vi "Sensor.vi"(0 "VISA resource name":refnum<visa-resource-name>, 7 "Channel (1)":i32=1 min=1 max=16 step=1, 11 "error in (no error)":errorcluster) -> (4 "VISA resource name out":refnum<visa-resource-name>, 6 "Resistance Reading":dbl min=0.0 max=63200000.0 step=1e-05 format="%^.5e", 8 "Kelvin Reading":dbl min=0.0 max=1000.0 step=1e-05 format="%^.5e", 10 "Power Reading":dbl min=0.0 max=0.01 step=1e-05 format="%^.5e", 15 "error out":errorcluster)   [LabVIEW 2014, in "Lake Shore Cryotronics 370.lvlib"]
doc: "This VI querys the instrument for an channels's sensor reading in Resistance, Kelvin, and Power."
uses:
  Lake Shore Cryotronics 370.lvlib
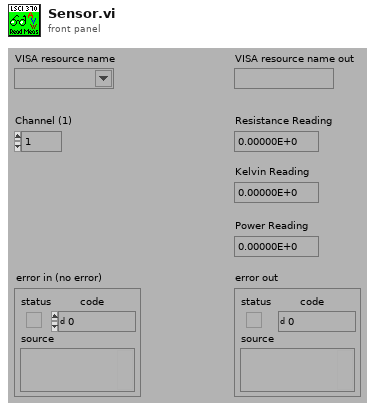
[diagram p1: front panel]
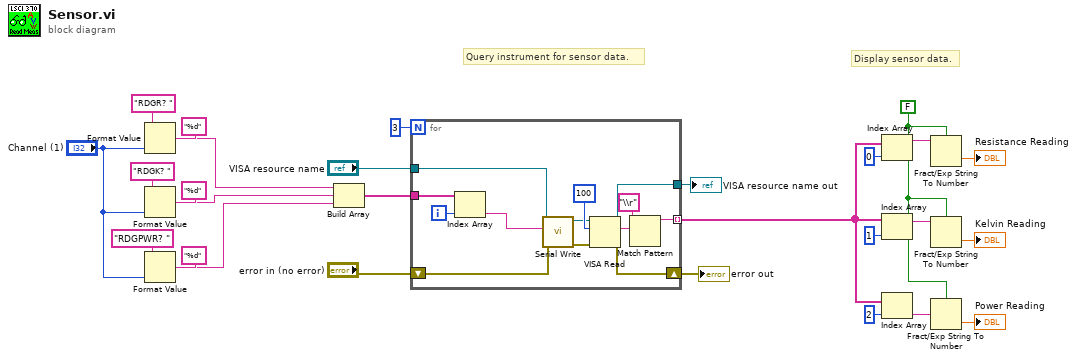
[diagram p0: block diagram]
diagram:
  w14 = FALSE ("use system decimal point (T)")
  # "Display sensor data."
  # "Query instrument for sensor data."
  n1 = Format Value(string ("")="RDGR? ", format string="%d", value (0)="Channel (1)") -> (output string=w6:string)
  n2 = Format Value(string ("")="RDGK? ", format string="%d", value (0)="Channel (1)") -> (output string=w5:string)
  n3 = Format Value(string ("")="RDGPWR? ", format string="%d", value (0)="Channel (1)") -> (output string=w4:string)
  n4 = Build Array(w6, w5, w4) -> (w21:string[])
  n5 = for {
    N: 3 -> [_]
    tunnel: w21 -> [w37]
    shift-right: [w34] -> w17
    shift-left: "error in (no error)" -> [w35]
    tunnel: [w33] -> w16
    tunnel: "VISA resource name" -> [w32]
    tunnel: [w30] -> w15 mode=indexing
    i -> [w36]
    n6 = Index Array(array=w37, index=w36) -> (element=w28:string)
    n7 = call "Serial Write.vi"("error in (no error)"=w35, "Write Buffer (\"\")"=w28, "VISA resource name"=w32) -> ("error out"=w40:errorcluster, "VISA resource name out"=w29:refnum<visa-resource-name>)  [unwired: 6 in, 1 out]
    n8 = VISA Read(VISA resource name=w29, byte count=100, error in (no error)=w40) -> (VISA resource name out=w33:refnum<visa-resource-name>, read buffer=w38:string, error out=w34:errorcluster)  [unwired: 1 out]
    n9 = Match Pattern(string=w38, regular expression="\\r") -> (before substring=w30:string)  [unwired: 1 in, 3 out]
  }
  "VISA resource name out" <- w16
  "error out" <- w17
  n10 = Index Array(array=w15, index=0) -> (element=w25:string)
  n11 = Index Array(array=w15, index=1) -> (element=w26:string)
  n12 = Index Array(array=w15, index=2) -> (element=w27:string)
  n13 = Fract/Exp String To Number(use system decimal point (T)=w14, string=w25) -> (number=→"Resistance Reading":dbl)  [unwired: 2 in, 1 out]
  n14 = Fract/Exp String To Number(use system decimal point (T)=w14, string=w26) -> (number=→"Kelvin Reading":dbl)  [unwired: 2 in, 1 out]
  n15 = Fract/Exp String To Number(use system decimal point (T)=w14, string=w27) -> (number=→"Power Reading":dbl)  [unwired: 2 in, 1 out]
